vi "9612 Invalid Value for PDO Mapping--error.vi"(8 "error in":errorcluster, 11 "PDO Mapping Value":u8) -> (0 "error out":errorcluster)   [LabVIEW 2024, in "Electronic Datasheet.lvlib"]
uses:
  Electronic Datasheet.lvlib
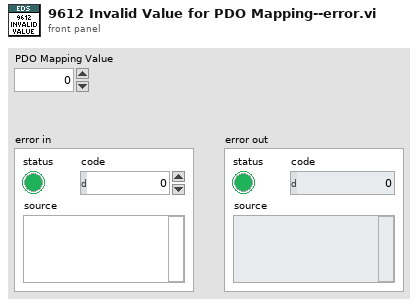
[diagram p1: front panel]
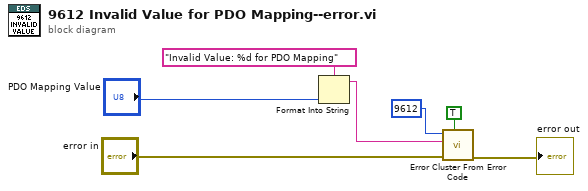
[diagram p0: block diagram]
diagram:
  n1 = Format Into String(format string="Invalid Value: %d for PDO Mapping", "PDO Mapping Value") -> (resulting string=w2:string)  [unwired: 2 in, 1 out]
  n2 = call <vilib>:"Error Cluster From Error Code.vi"("show call chain? (False)"=TRUE, "error in (no error)"="error in", "error message (\"\")"=w2, "error code (0)"=9612) -> ("error out"=→"error out":errorcluster)  [unwired: 5 in]
